vi "Ultrasonic PID.vi"(0 "refnum name":string="My Encoder RefNum", 1 "Enable? 2":bool, 2 "setpoint":dbl format="%.2f", 3 "X":dbl, 4 "Y":dbl) -> (5 "Enable?":bool, 6 "Y out":dbl, 7 "X out":dbl)   [LabVIEW 2013]
uses:
  <vilib>/addons/control/pid/pid.llb/PID (DBL).vi
  <vilib>/addons/control/pid/NI_PID_pid.lvlib
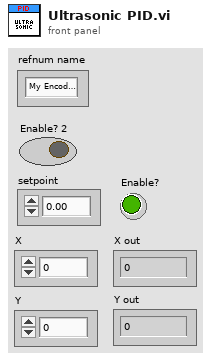
[diagram p1: front panel]
types:
  T1 = cluster{"proportional gain (Kc)":dbl, "integral time (Ti, min)":dbl, "derivative time (Td, min)":dbl}
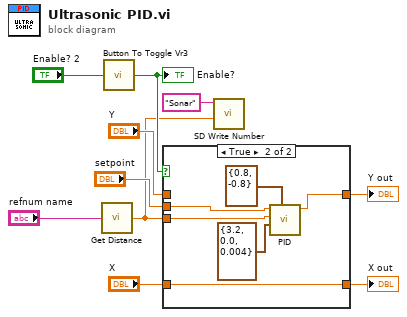
[diagram p0: block diagram]
diagram:
  n1 = call "Get Distance.vi"("refnum name"="refnum name") -> ("distance"=w2:dbl)
  n2 = call "Button To Toggle Vr3.vi"("InValue"="Enable? 2") -> ("Result"=w8:bool)
  "Enable?" <- w8
  n3 = case shown="True" w8 {
    tunnel: "setpoint" -> [_ w17]
    tunnel: [w12 w13] -> w4
    tunnel: [w11 w15] -> w7
    tunnel: "X" -> [w11 w15]
    tunnel: "Y" -> [w12 _]
    tunnel: w2 -> [_ w14]
    frame False {
    }
    frame True {
      n4 = call-poly <vilib>:"PID.vi"("output range"=cluster{"output high":dbl, "output low":dbl} {"output high"=0.8, "output low"=-0.8}, "PID gains"=T1 {"proportional gain (Kc)"=3.2, "integral time (Ti, min)"=0.0, "derivative time (Td, min)"=0.004}, "process variable"=w14, "setpoint"=w17) -> ("output"=w13:dbl)  [unwired: 6 in, 1 out]
    }
  }
  "X out" <- w7
  "Y out" <- w4
  n5 = call <vilib>:"SD Write Number.vi"("Numeric"=w2, "Name"="Sonar") -> ()  [unwired: 8 in, 2 out]
